vi "getResidue.vi"(8 "error in (no error)":errorcluster, 11 "LaguerreDeconEngineClass in":refnum<class "LaguerreDeconEngineClass.lvclass">) -> (0 "error out":errorcluster, 2 "R-square":dbl, 3 "LaguerreDeconEngineClass out":refnum<class "LaguerreDeconEngineClass.lvclass">, 4 "RMSE":dbl, 5 "SSE":dbl)   [LabVIEW 2020, in "LaguerreDeconEngineClass.lvclass"]
uses:
  LaguerreDeconEngineClass.lvclass
  LaguerreDeconEngineClass.lvclass/LaguerreDeconEngineClass.ctl
  <vilib>/Analysis/NI_AALPro.lvlib
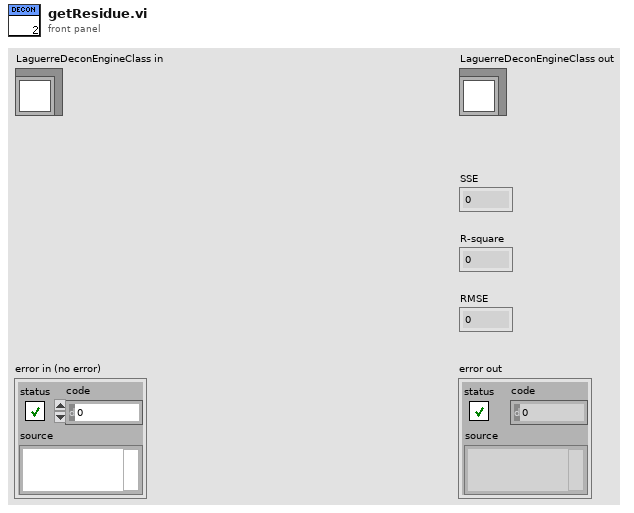
[diagram p1: front panel]
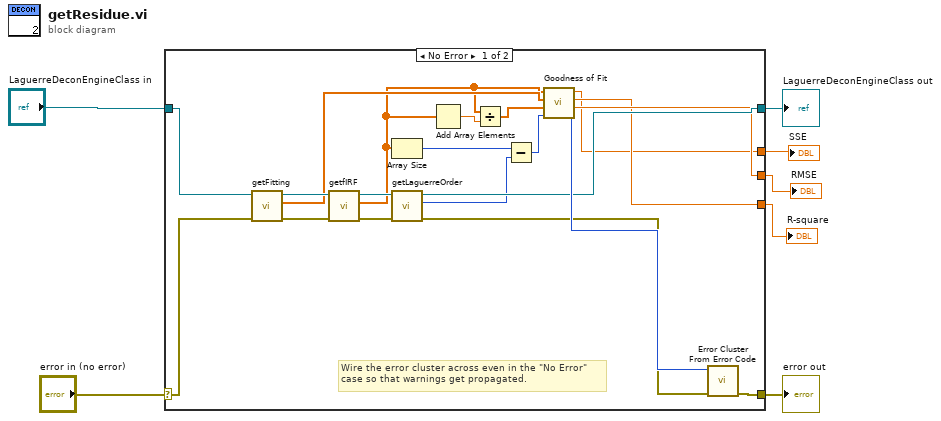
[diagram p0: block diagram]
diagram:
  n1 = case shown="No Error" "error in (no error)" {
    selector: "error in (no error)" -> [w24 w29]
    tunnel: [w22 w29] -> w6
    tunnel: [w20 w28] -> w4
    tunnel: "LaguerreDeconEngineClass in" -> [w27 w28]
    tunnel: [w13 _] -> w3
    tunnel: [w12 _] -> w2
    tunnel: [w11 _] -> w1
    frame No Error {
      # "Wire the error cluster across even in the \"No Error\"\ncase so that warnings get propagated."
      n2 = call "getFitting.vi"("error in (no error)"=w24, "LaguerreDeconEngineClass in"=w27) -> ("error out"=w25:errorcluster, "Fitting"=w17:dbl[], "LaguerreDeconEngineClass out"=w26:refnum<class "LaguerreDeconEngineClass.lvclass">)  [unwired: 7 in]
      n3 = call "getfIRF.vi"("error in (no error)"=w25, "LaguerreDeconEngineClass in"=w26) -> ("error out"=w19:errorcluster, "fIRF"=w10:dbl[], "LaguerreDeconEngineClass out"=w21:refnum<class "LaguerreDeconEngineClass.lvclass">)  [unwired: 7 in]
      n4 = Array Size(array=w10) -> (size(s)=w16:i32)
      n5 = call "getLaguerreOrder.vi"("error in (no error)"=w19, "LaguerreDeconEngineClass in"=w21) -> ("error out"=w18:errorcluster, "LaguerreOrder"=w15:u32, "LaguerreDeconEngineClass out"=w20:refnum<class "LaguerreDeconEngineClass.lvclass">)  [unwired: 7 in]
      n6 = Add Array Elements(numeric array=w10) -> (sum=w9:dbl)
      n7 = Divide(x=w10, y=w9) -> (x/y=w8:dbl[])
      n8 = Subtract(x=w16, y=w15) -> (x-y=w14:u32)
      n9 = call <vilib>:"Goodness of Fit.vi"("degree of freedom"=w14, "Weight"=w8, "Best Fit"=w17, "Y"=w10) -> ("error"=w23:i32, "RMSE"=w13:dbl, "R-square"=w12:dbl, "SSE"=w11:dbl)  [unwired: 4 in]
      n10 = call <vilib>:"Error Cluster From Error Code.vi"("error in (no error)"=w18, "error code (0)"=w23) -> ("error out"=w22:errorcluster)  [unwired: 7 in]
    }
    frame Error {
    }
  }
  "error out" <- w6
  "LaguerreDeconEngineClass out" <- w4
  "RMSE" <- w3
  "R-square" <- w2
  "SSE" <- w1
